vi "Cálculo de nsr.vi"(6 ">>tn>>":i32, 9 ">>n[]>>":csg[](array[numeric]), 10 "Tamaño (r)":i32, 11 ">>sr>>":cdb[](array[numeric])) -> (3 ">>nsr>>":cdb[](array[numeric]))   [LabVIEW 2013]
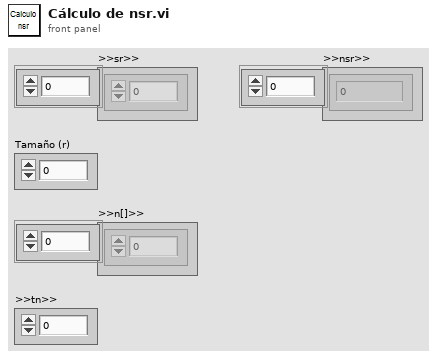
[diagram p1: front panel]
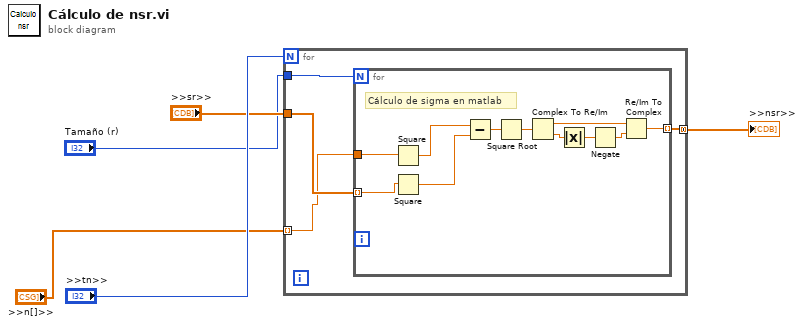
[diagram p0: block diagram]
diagram:
  n1 = for {
    N: ">>tn>>" -> [_]
    tunnel: "Tamaño (r)" -> [w9]
    tunnel: [w8] -> w4 mode=concatenating
    tunnel: ">>n[]>>" -> [w6] mode=indexing
    tunnel: ">>sr>>" -> [w7]
    n2 = for {
      N: w9 -> [_]
      tunnel: [w15] -> w8 mode=indexing
      tunnel: w7 -> [w11] mode=indexing
      tunnel: w6 -> [w10]
      # "Cálculo de sigma en matlab"
      n3 = Square(x=w10) -> (x^2=w13:csg)
      n4 = Square(x=w11) -> (x^2=w12:cdb)
      n5 = Subtract(x=w13, y=w12) -> (x-y=w20:cdb)
      n6 = Square Root(x=w20) -> (sqrt(x)=w14:cdb)
      n7 = Complex To Re/Im(x + iy=w14) -> (x=w19:dbl, y=w18:dbl)
      n8 = Absolute Value(x=w18) -> (abs(x)=w17:dbl)
      n9 = Negate(x=w17) -> (-x=w16:dbl)
      n10 = Re/Im To Complex(1:w16, 2:w19) -> (0:w15:cdb)
    }
  }
  ">>nsr>>" <- w4
